vi "Main.vi"(11 "Module Admin":refnum<class "Delacor_lib_QMH_Cloneable Module Admin.lvclass">) -> ()   [LabVIEW 2020, in "Graph Module.lvlib"]
doc: "This template is based off of the Queued Message Handler design pattern and the Queued Message Handler project template that ships with LabVIEW.\n\nThe main difference is that the queue is private to this module and communication between modules is performed via Broadcast and Request events.\n\nRequest events are wrapped in public API methods and are handled in the Event Handling Loop (EHL) of this VI. Any module can register for Broadcast events sent by this module. The EHL generates messages based on user interface actions.\n\nThe Message Handling Loop (MHL) processes messages generated by the EHL, or by other messages. The messages are string values, so new messages can be added easily to the Message Cases case structure in the MHL. Each message cluster can also provide an optional value for Message Data, which is a variant that can be converted to whatever message-specific data is required.\n_____\nBased on DQMH Project Template 6.0.0.91."
uses:
  Graph Module.lvlib
  <vilib>/Delacor/Delacor QMH/Libraries/Cloneable Module Admin_class/Delacor_lib_QMH_Cloneable Module Admin.lvclass
  C:/Program Files (x86)/National Instruments/LabVIEW 2020/vi.lib/Delacor/Delacor QMH/Libraries/Module Admin_class/Delacor_lib_QMH_Module Admin.lvclass
  Module Data--cluster.ctl
  <vilib>/Delacor/Delacor QMH/Libraries/Message Queue_class/Delacor_lib_QMH_Message Queue.lvclass/Delacor_lib_QMH_Message Queue.ctl
  <vilib>/Delacor/Delacor QMH/Libraries/Cloneable Module Admin_class/Delacor_lib_QMH_Cloneable Module Admin.lvclass/Delacor_lib_QMH_Cloneable Module Admin.ctl
  Stop Argument--cluster.ctl
  <vilib>/Delacor/Delacor QMH/Libraries/Module Admin_class/Delacor_lib_QMH_Module Admin.lvclass/Delacor_lib_QMH_Module Admin.ctl
  controls/commands.ctl
  controls/markerType.ctl
  Load DXF Argument--cluster.ctl
  Mark Coord Argument--cluster.ctl
  <vilib>/Delacor/Delacor QMH/Libraries/Message Queue_class/Delacor_lib_QMH_Enqueue Message (Single).vi
  <vilib>/Delacor/Delacor QMH/Libraries/Cloneable Module Admin_class/Delacor_lib_QMH_Get Module ID.vi
  <vilib>/Delacor/Delacor QMH/Libraries/Module Admin_class/Delacor_lib_QMH_Get External Launch.vi
  <vilib>/Utility/error.llb/Error Cluster From Error Code.vi
  <vilib>/ErrorRing/Error Ring.xnode
  <vilib>/Delacor/Delacor QMH/Libraries/Message Queue_class/Delacor_lib_QMH_Message Queue.lvclass
  Graph Extensions.lvlib
panel:
  out "XY Graph":cluster{dbl[], dbl[]}[](graph) caption="XY Graph - Light"
  out "error out":errorcluster
  out "Status":string
  in  "Simulate EHL Error":bool
  in  "Simulate MHL Error":bool
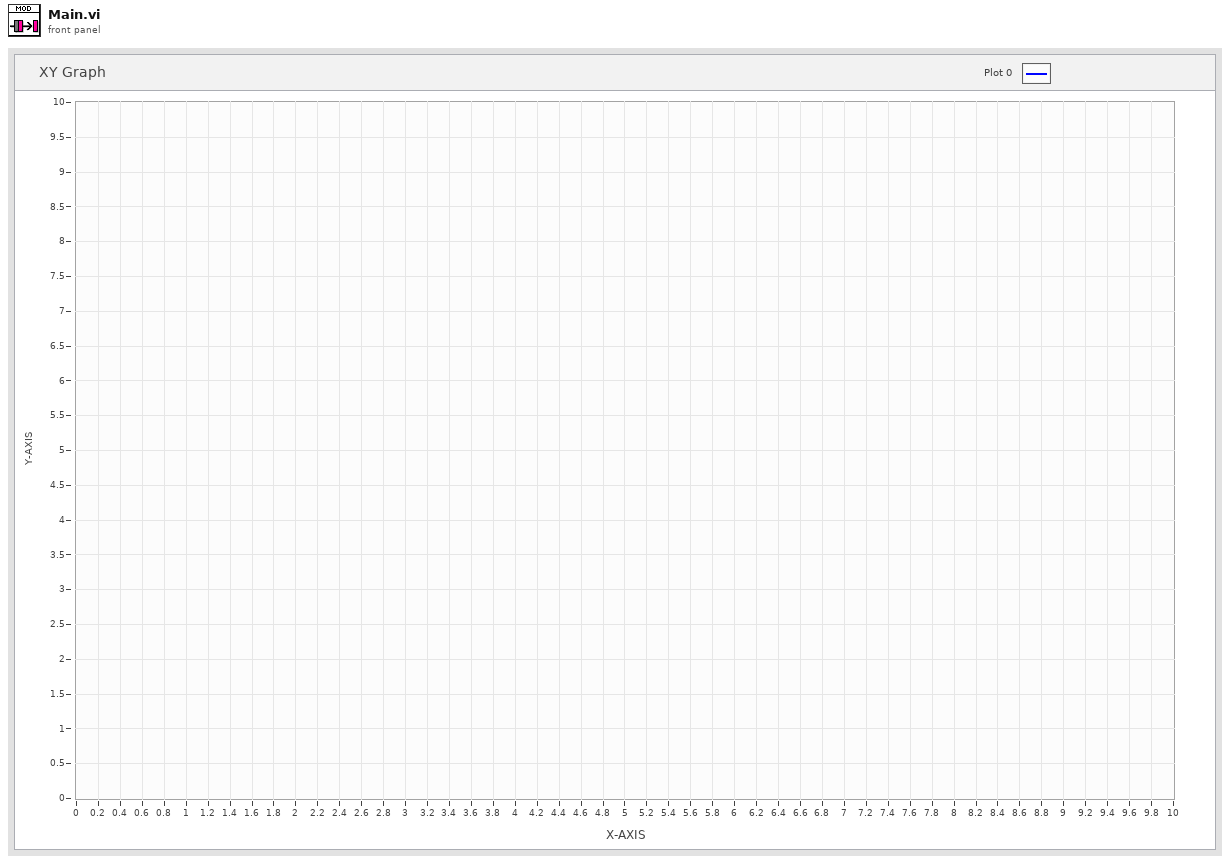
[diagram p1: front panel]
types:
  T1 = typedef "Graph Module.lvlib/Request Events--cluster.ctl" = cluster{"Stop Module":refnum<user-event>, "Show Panel":refnum<user-event>, "Hide Panel":refnum<user-event>, "Show Diagram":refnum<user-event>, "Get Module Execution Status":refnum<user-event>, "Load DXF":refnum<user-event>, "Mark Coord":refnum<user-event>}
  T2 = typedef "Graph Module.lvlib/Module Data--cluster.ctl" = cluster{"Status":string, "XY Graph":refnum<vi>}
  T3 = enum32{"invalid lock state", "Not Locked", "Locked (No Password)", "Password-protected"}
  T4 = typedef "Graph Module.lvlib/Stop Argument--cluster.ctl" = cluster{"Module ID":i32, "Origin":string, "Exit via Stop Module Req?":bool, "Wait for Module to stop?":bool}
  T5 = typedef "Graph Extensions.lvlib/commands.ctl" = enum16{"up", "options", "click", "move", "type", "redraw", "edited", "exit", "Mark"}
  T6 = typedef "Graph Extensions.lvlib/markerType.ctl" = enum16{"point", "arrow", "horiz", "vert", "vert range", "horiz range", "box"}
  T7 = typedef "Graph Module.lvlib/Load DXF Argument--cluster.ctl" = cluster{"Module ID":i32, "Path":path}
  T8 = typedef "Graph Module.lvlib/Mark Coord Argument--cluster.ctl" = cluster{"Module ID":i32, "XY Coord":cluster{"X":dbl, "Y":dbl}}
  T9 = enum32{"Invalid", "Standard", "Closed", "Hidden", "Minimized", "Maximized"}
  T10 = cluster{"Shift":bool, "Ctrl":bool, "Alt":bool, "Cmd":bool, "Opt":bool}
  T11 = typedef "LVPoint32TypeDef.ctl" = cluster{"Horizontal":i32, "Vertical":i32}
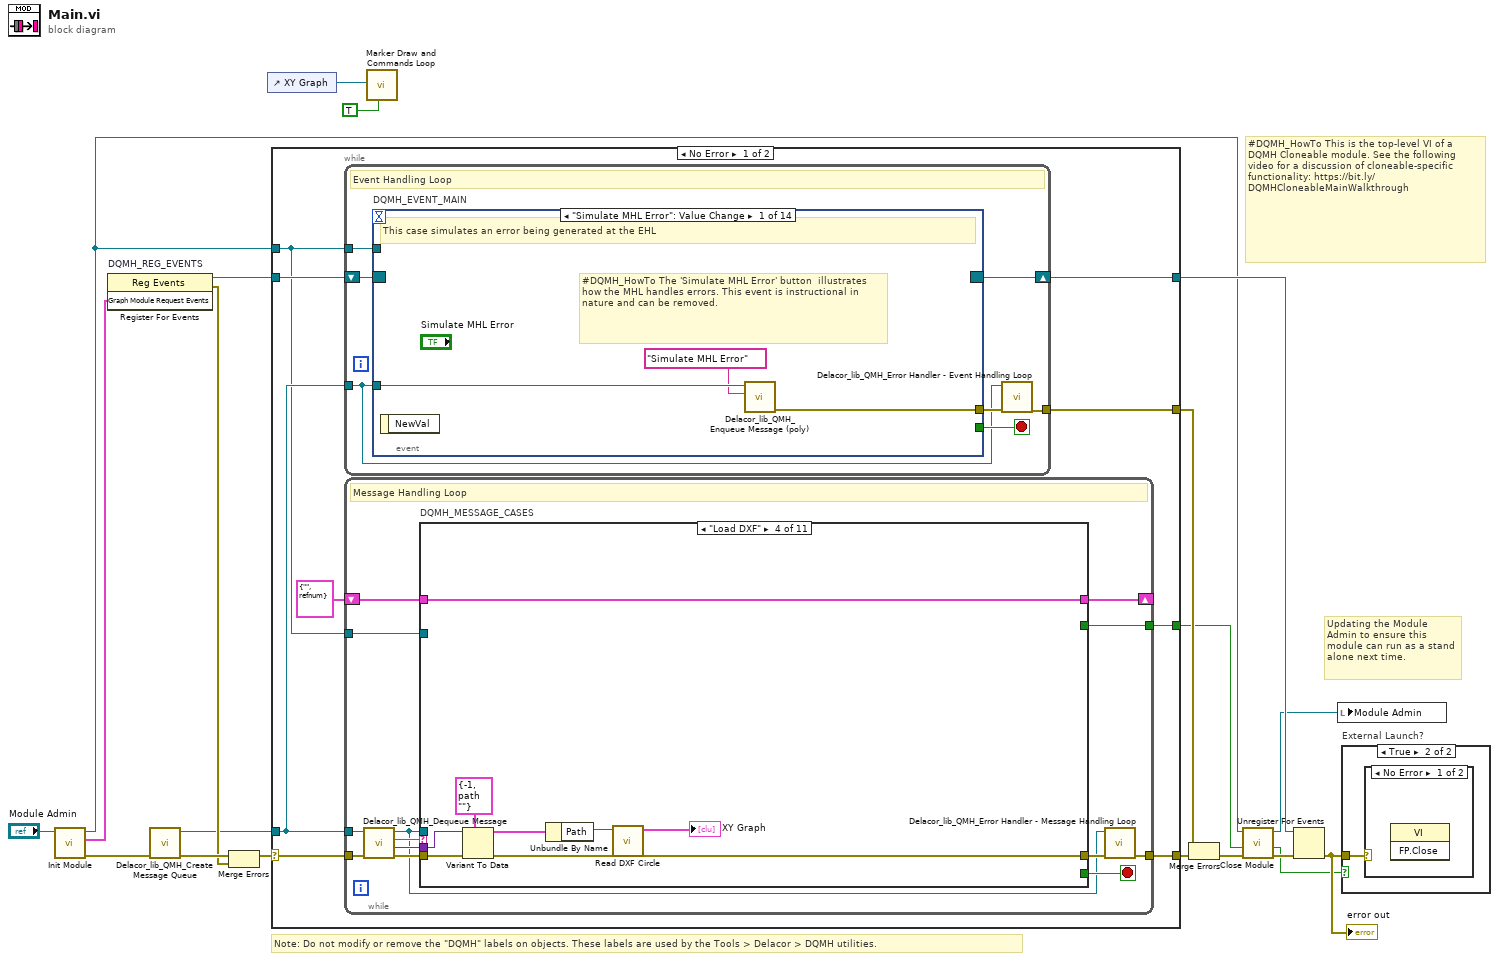
[diagram p0: block diagram]
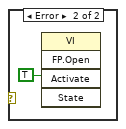
[diagram p3: hidden frame]
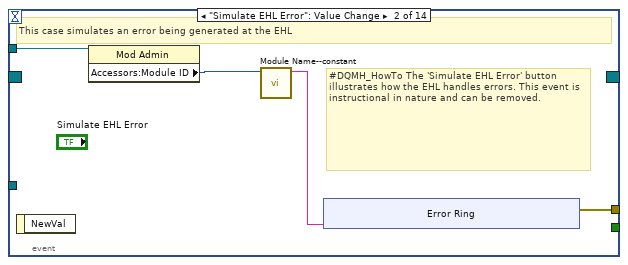
[diagram p4: hidden frame]
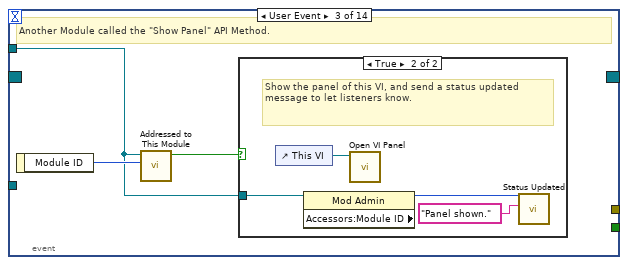
[diagram p5: hidden frame]
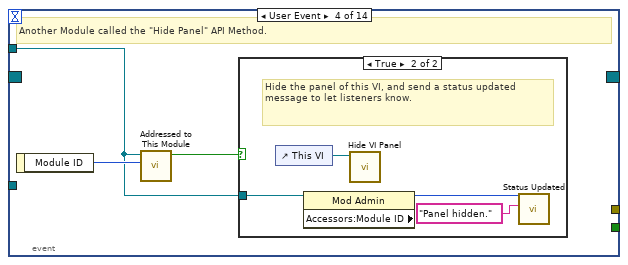
[diagram p7: hidden frame]
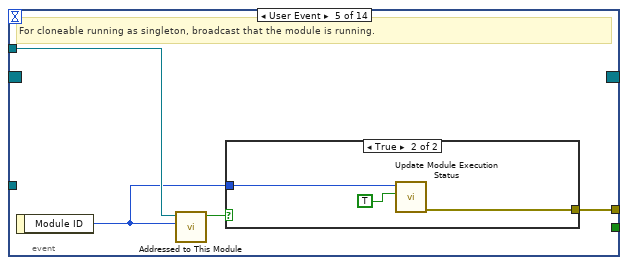
[diagram p9: hidden frame]
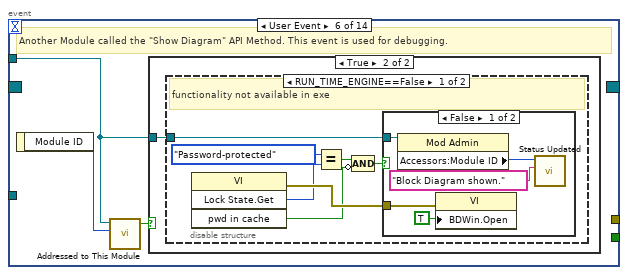
[diagram p11: hidden frame]
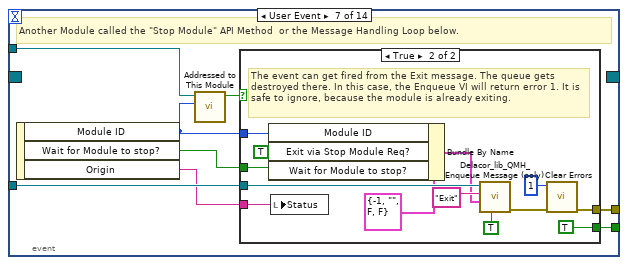
[diagram p15: hidden frame]
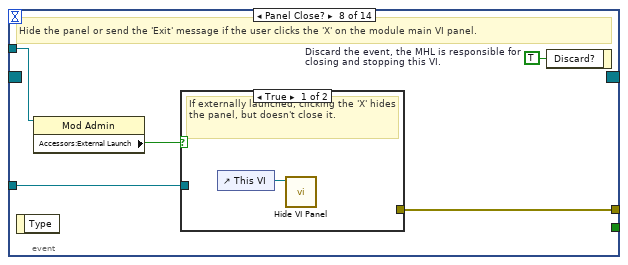
[diagram p17: hidden frame]
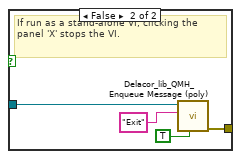
[diagram p18: hidden frame]
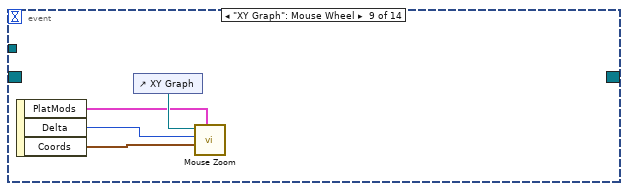
[diagram p19: hidden frame]
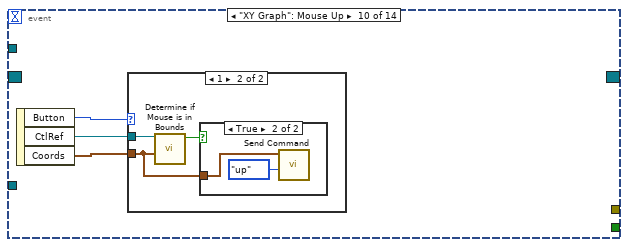
[diagram p20: hidden frame]
diagram:
  # "#DQMH_HowTo This is the top-level VI of a DQMH Cloneable module. See the following video for a discussion of cloneable-specific functionality: https://bit.ly/DQMHCloneableMainWalkthrough"
  # "Note: Do not modify or remove the \"DQMH\" labels on objects. These labels are used by the Tools > Delacor > DQMH utilities."
  # "Updating the Module Admin to ensure this module can run as a stand alone next time."
  n1 = call "Init Module.vi"("Cloneable Module Admin in"="Module Admin") -> ("error out"=w17:errorcluster, "Graph Module Request Events"=w9:T1, "Cloneable Module Admin out"=w6:refnum<class "Delacor_lib_QMH_Cloneable Module Admin.lvclass">)  [unwired: 8 in]
  n2 = register-events "DQMH_REG_EVENTS"(w9) -> (reference out=w10:refnum<event-registration>, error out=w12:errorcluster)  [unwired: 2 in]
  n3 = call <vilib>:"Delacor_lib_QMH_Create Message Queue.vi"("error in"=w17) -> ("error out"=w14:errorcluster, "Message Queue"=w8:refnum<class "Delacor_lib_QMH_Message Queue.lvclass">)  [unwired: 9 in]
  n4 = Merge Errors(w14, w12) -> (w13:errorcluster)
  n5 = control-ref of="XY Graph"() -> (w1:refnum<vi>)
  n6 = case shown="No Error" w13 {
    selector: w13 -> [w27 w322]
    tunnel: [w29 w321] -> w18
    tunnel: [w26 w329] -> w11
    tunnel: w10 -> [w24 w329]
    tunnel: w8 -> [w23 w320]
    tunnel: [w28 _] -> w19
    tunnel: w6 -> [w22 w325]
    tunnel: [w21 _] -> w4
    frame No Error {
      n7 = while {
        tunnel: w23 -> [w30]
        shift-right: [w33] -> w26
        shift-left: w24 -> [w34]
        tunnel: [w35] -> w28
        tunnel: w22 -> [w31]
        stop <- w32 stop-if-true
        # "Event Handling Loop"
        n8 = event "DQMH_EVENT_MAIN" shown="[0] \"Simulate MHL Error\": Value Change" {
          selector: w34 -> [_ _ _ _ _ _ _ _ _ _ _ _ _ _]
          dyn-events: [_ _ _ _ _ _ _ _ _ _ _ _ _ _] -> w33
          timeout: _ -> [_ _ _ _ _ _ _ _ _ _ _ _ _ _]
          tunnel: [_ _ _ _ _ _ w91 _ _ _ _ _ _ _] -> w32
          tunnel: w30 -> [w38 _ _ _ _ _ w94 w110 _ _ _ _ w171 w183]
          tunnel: [w39 w43 _ _ w68 _ w95 w113 _ _ w131 w154 w164 w176] -> w36
          tunnel: w31 -> [_ w42 w51 w58 w66 w72 w93 w111 _ _ w133 w156 w169 w181]
          event "Simulate MHL Error": Value Change {
            # "#DQMH_HowTo The 'Simulate MHL Error' button  illustrates how the MHL handles errors. This event is instructional in nature and can be removed."
            # "This case simulates an error being generated at the EHL"
            n9 = event-data() -> ()  [unwired: 1 in, 1 out]
            n10 = call-poly <vilib>:"Delacor_lib_QMH_Enqueue Message (poly).vi"("Message"="Simulate MHL Error", "Message Queue in"=w38) -> ("error out"=w39:errorcluster)  [unwired: 8 in, 1 out]
          }
          event "Simulate EHL Error": Value Change {
            # "#DQMH_HowTo The 'Simulate EHL Error' button  illustrates how the EHL handles errors. This event is instructional in nature and can be removed."
            # "This case simulates an error being generated at the EHL"
            n11 = event-data() -> ()  [unwired: 1 in, 1 out]
            n12 = property class="Mod Admin"(reference=w42) -> ("Accessors:Module ID"=w41:i32)  [unwired: 1 in, 2 out]
            n13 = call "Module Name--constant.vi"("Module ID"=w41) -> ("Module Name"=w40:string)  [unwired: 10 in]
            n14 = xnode "Error Ring"("parameter 0"=w40) -> ("error out"=w43:errorcluster)
          }
          event User Event {
            # "Another Module called the \"Show Panel\" API Method."
            n15 = event-data() -> ("Module ID"=w52:i32)  [unwired: 1 in]
            n16 = call "Addressed to This Module.vi"("Module ID from Argument"=w52, "Module Admin"=w51) -> ("Addressed to this instance?"=w53:bool)  [unwired: 8 in, 1 out]
            n17 = case shown="True" w53 {
              tunnel: w51 -> [_ w55]
              frame False {
              }
              frame True {
                # "Show the panel of this VI, and send a status updated message to let listeners know."
                n18 = control-ref of="This VI"() -> (w57:refnum<vi>)
                n19 = property class="Mod Admin"(reference=w55) -> ("Accessors:Module ID"=w54:i32)  [unwired: 1 in, 2 out]
                n20 = call "Open VI Panel.vi"("VI"=w57) -> ()  [unwired: 10 in, 1 out]
                n21 = call "Status Updated.vi"("Status"="Panel shown." ("format string"), "Module ID"=w54) -> ()  [unwired: 9 in, 1 out]
              }
            }
          }
          event User Event {
            # "Another Module called the \"Hide Panel\" API Method."
            n22 = event-data() -> ("Module ID"=w59:i32)  [unwired: 1 in]
            n23 = call "Addressed to This Module.vi"("Module ID from Argument"=w59, "Module Admin"=w58) -> ("Addressed to this instance?"=w60:bool)  [unwired: 8 in, 1 out]
            n24 = case shown="True" w60 {
              tunnel: w58 -> [_ w62]
              frame False {
              }
              frame True {
                # "Hide the panel of this VI, and send a status updated message to let listeners know."
                n25 = control-ref of="This VI"() -> (w64:refnum<vi>)
                n26 = property class="Mod Admin"(reference=w62) -> ("Accessors:Module ID"=w61:i32)  [unwired: 1 in, 2 out]
                n27 = call "Hide VI Panel.vi"("VI"=w64) -> ()  [unwired: 10 in, 1 out]
                n28 = call "Status Updated.vi"("Status"="Panel hidden." ("format string"), "Module ID"=w61) -> ()  [unwired: 9 in, 1 out]
              }
            }
          }
          event User Event {
            # "For cloneable running as singleton, broadcast that the module is running."
            n29 = event-data() -> ("Module ID"=w65:i32)  [unwired: 1 in]
            n30 = call "Addressed to This Module.vi"("Module ID from Argument"=w65, "Module Admin"=w66) -> ("Addressed to this instance?"=w67:bool)  [unwired: 8 in, 1 out]
            n31 = case shown="True" w67 {
              tunnel: [_ w71] -> w68
              tunnel: w65 -> [_ w70]
              frame False {
              }
              frame True {
                n32 = call "Update Module Execution Status.vi"("Running?"=TRUE, "Module ID"=w70) -> ("error out"=w71:errorcluster)  [unwired: 9 in]
              }
            }
          }
          event User Event {
            # "Another Module called the \"Show Diagram\" API Method. This event is used for debugging."
            n33 = event-data() -> ("Module ID"=w73:i32)  [unwired: 1 in]
            n34 = call "Addressed to This Module.vi"("Module ID from Argument"=w73, "Module Admin"=w72) -> ("Addressed to this instance?"=w74:bool)  [unwired: 8 in, 1 out]
            n35 = case shown="True" w74 {
              tunnel: w72 -> [_ w75]
              frame False {
              }
              frame True {
                n36 = disable-structure shown="RUN_TIME_ENGINE==False" {
                  disable-tunnel: w75 -> [w76 _]
                  frame condition #0 (active) {
                    # "functionality not available in exe"
                    n37 = invoke class="VI" method="Lock State.Get"() -> (error out=w82:errorcluster, "Get Lock State"=w81:T3, "pwd in cache"=w78:bool)  [unwired: 4 in, 1 out]
                    n38 = Equal?(x=T3."Password-protected", y=w81) -> (x = y?=w79:bool)
                    n39 = Compound Arithmetic op=AND(w79, invert w78) -> (w77:bool)
                    n40 = case shown="False" w77 {
                      tunnel: w82 -> [w87 _]
                      tunnel: w76 -> [w84 _]
                      frame False {
                        n41 = property class="Mod Admin"(reference=w84) -> ("Accessors:Module ID"=w83:i32)  [unwired: 1 in, 2 out]
                        n42 = property class="VI"(error in=w87, "BDWin.Open"=TRUE ("Block Diagram Window:Open")) -> ()  [unwired: 1 in, 2 out]
                        n43 = call "Status Updated.vi"("Status"="Block Diagram shown." ("format string"), "Module ID"=w83) -> ()  [unwired: 9 in, 1 out]
                      }
                      frame True {
                        # "Password-protected VI, and the password is not in the cache. Do not show the diagram."
                      }
                    }
                  }
                  frame condition #1 {
                  }
                }
              }
            }
          }
          event User Event {
            # "Another Module called the \"Stop Module\" API Method  or the Message Handling Loop below."
            n44 = event-data() -> ("Module ID"=w89:i32, "Wait for Module to stop?"=w90:bool, "Origin"=w88:string)  [unwired: 1 in]
            n45 = call "Addressed to This Module.vi"("Module ID from Argument"=w89, "Module Admin"=w93) -> ("Addressed to this instance?"=w92:bool)  [unwired: 8 in, 1 out]
            n46 = case shown="True" w92 {
              tunnel: [_ w107] -> w95
              tunnel: w94 -> [_ w103]
              tunnel: [_ TRUE] -> w91
              tunnel: w90 -> [_ w98]
              tunnel: w89 -> [_ w100]
              tunnel: w88 -> [_ w96]
              frame False {
              }
              frame True {
                # "The event can get fired from the Exit message. The queue gets destroyed there. In this case, the Enqueue VI will return error 1. It is safe to ignore, because the module is already exiting."
                n47 = Bundle By Name(cluster=T4 {"Module ID"=-1, "Origin"="", "Exit via Stop Module Req?"=FALSE, "Wait for Module to stop?"=FALSE} ("Stop Argument"), "Module ID"=w100, "Exit via Stop Module Req?"=TRUE, "Wait for Module to stop?"=w98) -> (w97:T4)
                n48 = local write "Status"(w96) -> ()
                n49 = call-poly <vilib>:"Delacor_lib_QMH_Enqueue Message (poly).vi"("Priority Message? (F)"=TRUE, "Message Data"=w97, "Message"="Exit", "Message Queue in"=w103) -> ("error out"=w108:errorcluster)  [unwired: 6 in, 1 out]
                n50 = call <vilib>:"Clear Errors.vi"("error in (no error)"=w108, "specific error code to clear (0: all)"=1) -> ("error out"=w107:errorcluster)  [unwired: 4 in, 1 out]
              }
            }
          }
          event Panel Close? {
            w112 = TRUE  # Discard the event, the MHL is responsible for closing and stopping this VI.
            # "Hide the panel or send the 'Exit' message if the user clicks the 'X' on the module main VI panel."
            n51 = event-data() -> ()  [unwired: 1 in, 1 out]
            n52 = property class="Mod Admin"(reference=w111) -> ("Accessors:External Launch"=w109:bool)  [unwired: 1 in, 2 out]
            n53 = case shown="True" w109 {
              tunnel: w110 -> [_ w117]
              tunnel: [_ w118] -> w113
              frame True {
                # "If externally launched, clicking the 'X' hides the panel, but doesn't close it."
                n54 = control-ref of="This VI"() -> (w114:refnum<vi>)
                n55 = call "Hide VI Panel.vi"("VI"=w114) -> ()  [unwired: 10 in, 1 out]
              }
              frame False {
                # "If run as a stand-alone VI, clicking the panel 'X' stops the VI."
                n56 = call-poly <vilib>:"Delacor_lib_QMH_Enqueue Message (poly).vi"("Priority Message? (F)"=TRUE, "Message"="Exit", "Message Queue in"=w117) -> ("error out"=w118:errorcluster)  [unwired: 7 in, 1 out]
              }
            }
            n57 = event-data("Discard?"=w112) -> ()  [unwired: 1 in, 1 out]
          }
          event "XY Graph": Mouse Wheel {
            n58 = event-data() -> ("PlatMods"=w119:T10, "Delta"=w121:i32, "Coords"=w120:T11)  [unwired: 1 in]
            n59 = control-ref of="XY Graph"() -> (w122:refnum<vi>)
            n60 = call "Mouse Zoom.vi"("PlatMods"=w119, "XY"=w120, "Delta"=w121, "XY Graph"=w122) -> ()  [unwired: 8 in]
          }
          event "XY Graph": Mouse Up {
            n61 = event-data() -> ("Button"=w123:u16, "CtlRef"=w124:refnum<vi>, "Coords"=w125:T11)  [unwired: 1 in]
            n62 = case shown="1" w123 {
              tunnel: w125 -> [_ w127]
              tunnel: w124 -> [_ w128]
              frame Default {
              }
              frame 1 {
                n63 = call "Determine if Mouse is in Bounds.vi"("Coords"=w127, "XYGraph in"=w128) -> ("In bounds?"=w126:bool)  [unwired: 9 in]
                n64 = case shown="True" w126 {
                  tunnel: w127 -> [_ w129]
                  frame False {
                  }
                  frame True {
                    n65 = call "Send Command.vi"("cmd"=commands."up", "Coords"=w129) -> ()  [unwired: 10 in]
                  }
                }
              }
            }
          }
          event "XY Graph": Mouse Down {
            n66 = event-data() -> ("CtlRef"=w136:refnum<vi>, "Coords"=w135:T11, "Button"=w134:u16)  [unwired: 1 in]
            n67 = property class="Mod Admin"(reference=w133) -> ("Accessors:Module ID"=w132:i32)  [unwired: 1 in, 2 out]
            n68 = case shown="1" w134 {
              tunnel: w135 -> [_ w139 w148]
              tunnel: w136 -> [_ w138 w149]
              tunnel: w132 -> [_ _ w146]
              tunnel: [_ _ w145] -> w131
              frame Default {
              }
              frame 2 {
                n69 = call "Determine if Mouse is in Bounds.vi"("Coords"=w139, "XYGraph in"=w138) -> ("In bounds?"=w137:bool)  [unwired: 9 in]
                n70 = case shown="True" w137 {
                  frame False {
                  }
                  frame True {
                    n71 = call "Marker Types.vi"() -> ("Close"=w141:bool, "Type"=w140:T6)  [unwired: 10 in]
                    n72 = case shown="False" w141 {
                      tunnel: w140 -> [w143 _]
                      frame False {
                        n73 = call "Send Command.vi"("cmd"=commands."type", "Type"=w143) -> ()  [unwired: 10 in]
                      }
                      frame True {
                        n74 = call "Send Command.vi"("cmd"=commands."redraw") -> ()  [unwired: 11 in]
                      }
                    }
                  }
                }
              }
              frame 1 {
                n75 = call "Determine if Mouse is in Bounds.vi"("Coords"=w148, "XYGraph in"=w149) -> ("In bounds?"=w147:bool)  [unwired: 9 in]
                n76 = case shown="True" w147 {
                  tunnel: w148 -> [_ w150]
                  tunnel: w146 -> [_ w152]
                  tunnel: [_ w151] -> w145
                  frame False {
                  }
                  frame True {
                    n77 = invoke on="XY Graph" class="XYGraph (strict)" method="Map Coords To XY"("Coords"=w150) -> ("XY"=w153:cluster{"X":dbl, "Y":dbl})  [unwired: 6 in, 6 out]
                    n78 = call "Broadcast Coord.vi"("XY Coord"=w153, "Module ID"=w152) -> ("error out"=w151:errorcluster)  [unwired: 9 in]
                  }
                }
              }
            }
          }
          event "XY Graph": Mouse Move {
            n79 = event-data() -> ("Coords"=w157:T11)  [unwired: 1 in, 1 out]
            n80 = property class="Mod Admin"(reference=w156) -> ("Accessors:Module ID"=w155:i32)  [unwired: 1 in, 2 out]
            n81 = call "Send Command.vi"("cmd"=commands."move", "Type"=markerType."vert", "Coords"=w157) -> ()  [unwired: 9 in]
            n82 = disable-structure shown="Disabled" {
              disable-tunnel: w157 -> [w163 _]
              disable-tunnel: w155 -> [w161 _]
              disable-tunnel: [w160 _] -> w154
              frame Disabled {
                n83 = invoke on="XY Graph" class="XYGraph (strict)" method="Map Coords To XY"("Coords"=w163) -> ("XY"=w162:cluster{"X":dbl, "Y":dbl})  [unwired: 6 in, 6 out]
                n84 = call "Broadcast Coord.vi"("XY Coord"=w162, "Module ID"=w161) -> ("error out"=w160:errorcluster)  [unwired: 9 in]
              }
              frame Enabled {
              }
            }
          }
          event User Event {
            # "Another Module called the \"Load DXF\" API Method."
            n85 = event-data() -> ("Module ID"=w166:i32, "Path"=w165:path)  [unwired: 1 in]
            n86 = Bundle(cluster=T7 {"Module ID"=-1, "Path"=path ""} ("Load DXF Argument"), "Module ID"=w166, "Path"=w165) -> (w167:T7)
            n87 = call "Addressed to This Module.vi"("Module ID from Argument"=w166, "Module Admin"=w169) -> ("Addressed to this instance?"=w170:bool)  [unwired: 8 in, 1 out]
            n88 = case shown="True" w170 {
              tunnel: w171 -> [_ w175]
              tunnel: w167 -> [_ w173]
              tunnel: [_ w172] -> w164
              frame False {
              }
              frame True {
                n89 = call-poly <vilib>:"Delacor_lib_QMH_Enqueue Message (poly).vi"("Message Data"=w173, "Message"="Load DXF", "Message Queue in"=w175) -> ("error out"=w172:errorcluster)  [unwired: 7 in, 1 out]
              }
            }
          }
          event User Event {
            # "Another Module called the \"Mark Coord\" API Method."
            n90 = event-data() -> ("Module ID"=w178:i32, "XY Coord"=w177:cluster{"X":dbl, "Y":dbl})  [unwired: 1 in]
            n91 = Bundle(cluster=T8 {"Module ID"=-1, "XY Coord"={"X"=0.0, "Y"=0.0}} ("Mark Coord Argument"), "Module ID"=w178, "XY Coord"=w177) -> (w179:T8)
            n92 = call "Addressed to This Module.vi"("Module ID from Argument"=w178, "Module Admin"=w181) -> ("Addressed to this instance?"=w182:bool)  [unwired: 8 in, 1 out]
            n93 = case shown="True" w182 {
              tunnel: w183 -> [_ w187]
              tunnel: w179 -> [_ w185]
              tunnel: [_ w184] -> w176
              frame False {
              }
              frame True {
                n94 = call-poly <vilib>:"Delacor_lib_QMH_Enqueue Message (poly).vi"("Message Data"=w185, "Message"="Mark Coord", "Message Queue in"=w187) -> ("error out"=w184:errorcluster)  [unwired: 7 in, 1 out]
              }
            }
          }
        }
        n95 = call-dynamic "Delacor_lib_QMH_Error Handler - Event Handling Loop.vi"("error in"=w36, "Message Queue in"=w30) -> ("dup error in"=w35:errorcluster)  [unwired: 8 in, 1 out]
      }
      n96 = while {
        tunnel: w23 -> [w191]
        shift-right: [w195] -> _
        shift-left: T2 {"Status"="", "XY Graph"=refnum} ("Data Cluster") -> [w196]
        tunnel: w27 -> [w199]
        tunnel: [w197] -> w29
        tunnel: w22 -> [w189]
        tunnel: [w188] -> w21
        stop <- w194 stop-if-true
        # "Message Handling Loop"
        n97 = call-dynamic "Delacor_lib_QMH_Dequeue Message.vi"("error in"=w199, "Message Queue in"=w191) -> ("error out"=w198:errorcluster, "Message Data"=w192:variant, "Message"=w193:string, "Message Queue out"=w190:refnum<class "Delacor_lib_QMH_Message Queue.lvclass">)  [unwired: 6 in]
        n98 = case "DQMH_MESSAGE_CASES" shown="\"Load DXF\"" w193 {
          selector: w193 -> [_ _ _ _ _ _ _ _ _ _ w307]
          tunnel: w190 -> [w203 _ _ _ _ _ _ w257 _ w297 _]
          tunnel: w198 -> [w222 w226 w230 w239 w250 w253 w255 w266 w279 w303 w309]
          tunnel: [w221 w226 w230 w233 w240 w252 w255 w262 w278 w300 w310] -> w200
          tunnel: w196 -> [w214 w225 w229 w238 w249 w251 w254 w261 w276 w296 w308]
          tunnel: [w213 w225 w229 w238 w249 w251 w254 w261 w276 w296 w308] -> w195
          tunnel: [_ _ _ _ _ _ _ _ _ w295 _] -> w194
          tunnel: w192 -> [_ _ _ w237 w248 _ _ w260 _ w293 _]
          tunnel: w189 -> [w208 _ _ _ _ _ _ w259 w274 w289 w305]
          tunnel: [_ _ _ _ _ _ _ _ _ w291 _] -> w188
          frame "Initialize" {
            w206 = "Initial Message" ("Initial Message")
            # "#CodeNeeded - Initialize the appearance of the front panel."
            # "Initialize - Any operation that needs to be done before the module can receive messages. Synchronize Caller Events.vi will inform Start Module.vi that the module has launched and is ready to receive messages. Module Did Init.vi will broadcast that the module initialized."
            n99 = call "Synchronize Caller Events.vi"("error in (no error)"=w222, "Module Admin"=w208) -> ("error out"=w202:errorcluster, "Module Admin out"=w207:refnum<class "Delacor_lib_QMH_Cloneable Module Admin.lvclass">)  [unwired: 8 in]
            n100 = property class="Mod Admin"(reference=w207) -> ("Accessors:Module ID"=w210:i32, "Accessors:External Launch"=w209:bool)  [unwired: 1 in, 2 out]
            n101 = call "Module Name--constant.vi"("Module ID"=w210) -> ("Module Name"=w218:string)  [unwired: 10 in]
            n102 = control-ref of="XY Graph"() -> (w205:refnum<vi>)
            n103 = call-poly <vilib>:"Delacor_lib_QMH_Enqueue Message (poly).vi"("error in"=w202, "Message"="Initialize XY Graph", "Message Queue in"=w203) -> ("error out"=w201:errorcluster)  [unwired: 7 in, 1 out]
            n104 = property class="VI"("Front Panel.Title"=w218) -> (reference out=w220:refnum<vi>, error out=w224:errorcluster)  [unwired: 2 in]
            n105 = Select(t=T9."Hidden" ("State"), s=w209, f=T9."Standard" ("State")) -> (s? t:f=w215:T9)
            n106 = invoke class="VI" method="FP.Open"(reference=w220, error in=w224, "State"=w215) -> (reference out=w219:refnum<vi>, error out=w223:errorcluster)  [unwired: 2 in, 3 out]
            n107 = Bundle By Name(cluster=w214, "XY Graph"=w205, "Status"=w206) -> (w213:T2)
            n108 = call "Module Name--constant.vi"("Module ID"=w210) -> ("Module Name"=w211:string)  [unwired: 10 in]
            n109 = invoke class="VI" method="FP.Center"(reference=w219, error in=w223) -> ()  [unwired: 1 in, 3 out]
            n110 = call "Module Did Init.vi"("error in (no error)"=w201, "Initialized?"=TRUE, "Origin"=w211, "Module ID"=w210) -> ("error out"=w221:errorcluster)  [unwired: 7 in]
            "Status" <- w206
          }
          frame "---Module Specific---" {
            # "Separator -- The following cases handle messages specific to this Module."
          }
          frame "Initialize XY Graph" {
            n111 = Unbundle By Name(w229) -> ("XY Graph"=w227:refnum<vi>)
            n112 = property on="Property Node" class="XYGraph (strict)"(reference=w227, "ActPaletteTool"=0 ("Palette:Active Tool")) -> ()  [unwired: 1 in, 2 out]
          }
          frame "Load DXF" {
            n113 = Variant To Data(error in=w239, type=T7 {"Module ID"=-1, "Path"=path ""} ("Load DXF Argument"), Variant=w237) -> (data=w235:T7, error out=w234:errorcluster)
            n114 = Unbundle By Name(w235) -> ("Path"=w232:path)
            n115 = call "Read DXF Circle.vi"("error in (no error)"=w234, "path"=w232) -> ("error out"=w233:errorcluster, "XY graph"=→"XY Graph":cluster{dbl[], dbl[]}[])  [unwired: 5 in, 3 out]
          }
          frame "Mark Coord" {
            n116 = Variant To Data(error in=w250, type=T8 {"Module ID"=-1, "XY Coord"={"X"=0.0, "Y"=0.0}} ("Mark Coord Argument"), Variant=w248) -> (data=w246:T8, error out=w241:errorcluster)
            n117 = Unbundle By Name(w246) -> ("XY Coord"=w243:cluster{"X":dbl, "Y":dbl})
            n118 = invoke on="XY Graph" class="XYGraph (strict)" method="Map XY To Coords"(error in=w241, "XY"=w243) -> (error out=w240:errorcluster, "Coords"=w242:T11)  [unwired: 5 in, 5 out]
            n119 = call "Send Command.vi"("cmd"=commands."Mark", "Type"=markerType."vert", "Coords"=w242) -> ()  [unwired: 9 in]
          }
          frame "---Copy This Frame---" {
            # "Duplicate this frame when creating new messages.  Change this comment in the duplicated frame to describe this message."
            n120 = Merge Errors(w253) -> (w252:errorcluster)
          }
          frame "---Exit and Error Handling---" {
            # "Separator - the following cases handle errors and exit messages."
          }
          frame "Error" {
            # "#CodeRecommended - If you ever change the name of this \"Error\" message, you'll need to update the name in the Check Loop Error.vi as well."
            # "#CodeRecommended - If the module is running in standalone mode (External Launch = FALSE), this code will pop up an error dialog and call the 'Exit' message if an error occurs. Add more fine-grained error handling here."
            # "Error - Check the error message data and respond accordingly. This message is sent by the \"Error Handler\" VIs at the end of each loop in this application."
            n121 = Variant To Data(error in=w266, type=errorcluster {"status"=FALSE, "code"=0, "source"=""} ("error constant"), Variant=w260) -> (data=w267:errorcluster, error out=w264:errorcluster)
            n122 = property class="Mod Admin"(reference=w259) -> ("Accessors:External Launch"=w258:bool, "Accessors:Module ID"=w256:i32)  [unwired: 1 in, 2 out]
            n123 = call "Error Reported.vi"("Error"=w267, "Module ID"=w256) -> ()  [unwired: 9 in, 1 out]
            n124 = case shown="False" w258 {
              tunnel: [w272 _] -> w263
              tunnel: w257 -> [w270 _]
              tunnel: w267 -> [w271 _]
              frame False {
                # "If the module is running standalone, then pop up an error dialog and call the \"Exit\" message."
                n125 = call <vilib>:"Simple Error Handler.vi"("error in (no error)"=w271) -> ()  [unwired: 4 in, 5 out]
                n126 = call-poly <vilib>:"Delacor_lib_QMH_Enqueue Message (poly).vi"("Priority Message? (F)"=TRUE, "Message"="Exit", "Message Queue in"=w270) -> ("error out"=w272:errorcluster)  [unwired: 7 in, 1 out]
              }
              frame True {
                # "If the module was launched externally, calling the Error Reported broadcast VI is the only action performed by the \"Error\" message. The module's caller can then process the error appropriately."
              }
            }
            n127 = Merge Errors(w264, w263) -> (w262:errorcluster)
            n128 = local write "error out"(w262) -> ()
          }
          frame "Simulate MHL Error" {
            # "#DQMH_HowTo The 'Simulate MHL Error' button  illustrates how the MHL handles errors. This event is instructional in nature and can be removed."
            # "Simulate an error occurring at the MHL"
            n129 = property class="Mod Admin"(reference=w274) -> ("Accessors:Module ID"=w275:i32)  [unwired: 1 in, 2 out]
            n130 = call "Module Name--constant.vi"("Module ID"=w275) -> ("Module Name"=w273:string)  [unwired: 10 in]
            n131 = xnode "Error Ring"("parameter 0"=w273) -> ("error out"=w277:errorcluster)
            n132 = Merge Errors(w279, w277) -> (w278:errorcluster)
          }
          frame "Exit" {
            w294 = 91  # 91: not all Exit messages will have an argument
            w295 = TRUE  # Stop the VI
            # "Release the message queue reference"
            # "#CodeNeeded - Add any required cleanup code here."
            # "Exit - Exit the application."
            n133 = Variant To Data(error in=w303, type=T4 {"Module ID"=-1, "Origin"="", "Exit via Stop Module Req?"=FALSE, "Wait for Module to stop?"=FALSE} ("Stop Argument"), Variant=w293) -> (data=w290:T4, error out=w298:errorcluster)
            n134 = call <vilib>:"Clear Errors.vi"("error in (no error)"=w298, "specific error code to clear (0: all)"=w294) -> ("error out"=w302:errorcluster)  [unwired: 4 in, 1 out]
            n135 = control-ref of="This VI"() -> (w288:refnum<vi>)
            n136 = call-dynamic "Delacor_lib_QMH_Release Message Queue.vi"("error in"=w302, "Message Queue"=w297) -> ("error out"=w301:errorcluster)  [unwired: 9 in]
            n137 = call "Handle Exit.vi"("Stop Argument"=w290, "Module Admin in"=w289, "VI reference"=w288) -> ("error out"=w299:errorcluster, "Wait for Stop?"=w291:bool)  [unwired: 7 in]
            n138 = Merge Errors(w301, w299) -> (w300:errorcluster)
            n139 = call "Send Command.vi"("cmd"=commands."exit") -> ()  [unwired: 11 in]
          }
          frame Default {
            # "'Default' case only runs if there is a message that isn't defined in any of the other cases.  Output a programming error."
            n140 = property class="Mod Admin"(reference=w305) -> ("Accessors:Module ID"=w304:i32)  [unwired: 1 in, 2 out]
            n141 = call "Module Name--constant.vi"("Module ID"=w304) -> ("Module Name"=w306:string)  [unwired: 10 in]
            n142 = xnode "Error Ring"("parameter 0"=w307, "parameter 1"=w306) -> ("error out"=w311:errorcluster)
            n143 = Merge Errors(w309, w311) -> (w310:errorcluster)
          }
        }
        n144 = call-dynamic "Delacor_lib_QMH_Error Handler - Message Handling Loop.vi"("error in"=w200, "Message Queue in"=w190) -> ("dup error in"=w197:errorcluster)  [unwired: 8 in, 1 out]
      }
    }
    frame Error {
      n145 = call "Synchronize Caller Events.vi"("Module Admin"=w325) -> ("Module Admin out"=w324:refnum<class "Delacor_lib_QMH_Cloneable Module Admin.lvclass">)  [unwired: 9 in, 1 out]
      n146 = property class="Mod Admin"(reference=w324) -> ("Accessors:Module ID"=w323:i32)  [unwired: 1 in, 2 out]
      n147 = call-dynamic "Delacor_lib_QMH_Release Message Queue.vi"("error in"=w322, "Message Queue"=w320) -> ("error out"=w321:errorcluster)  [unwired: 9 in]
      n148 = call "Module Name--constant.vi"("Module ID"=w323) -> ("Module Name"=w328:string)  [unwired: 10 in]
      n149 = Format Into String(format string="An error occurred during initialization. %s is no longer running.", w328) -> (resulting string=w326:string)  [unwired: 2 in, 1 out]
      n150 = call "Error Reported.vi"("Additional Information"=w326, "Error"=w321, "Module ID"=w323) -> ()  [unwired: 8 in, 1 out]
    }
  }
  n151 = call "Marker Draw and Commands Loop.vi"("Enable Cursors"=TRUE, "XY Graph"=w1) -> ()  [unwired: 10 in]
  n152 = Merge Errors(w19, w18) -> (w20:errorcluster)
  n153 = call "Close Module.vi"("error in"=w20, "Wait for stop?"=w4, "Module Admin in"=w6) -> ("error out"=w16:errorcluster, "External Launch"=w3:bool, "Module Admin out"=w5:refnum<class "Delacor_lib_QMH_Cloneable Module Admin.lvclass">)  [unwired: 6 in]
  n154 = Unregister For Events(event registration refnum=w11, error in=w16) -> (error out=w15:errorcluster)
  "error out" <- w15
  n155 = local write "Module Admin"(w5) -> ()
  n156 = case "External Launch?" shown="True" w3 {
    tunnel: w15 -> [_ w330]
    frame False {
    }
    frame True {
      n157 = case shown="No Error" w330 {
        frame No Error {
          n158 = invoke class="VI" method="FP.Close"() -> ()  [unwired: 3 in, 3 out]
        }
        frame Error {
          n159 = invoke class="VI" method="FP.Open"("Activate"=TRUE ("Activate?")) -> ()  [unwired: 4 in, 5 out]
        }
      }
    }
  }
